vi "Bump Turret Az.vi"() -> ()   [LabVIEW 2016]
panel:
  in  "D-Pad":T1(radio)
  in  "reset":bool
  out "offset":dbl
  out "arctan(x)":dbl
  in  "D":dbl
  in  "d":dbl
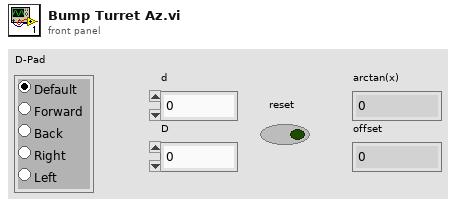
[diagram p1: front panel]
types:
  T1 = enum32{"Default", "Radio Selection 2", "Radio Selection 4", "Radio Selection 3", "Radio Selection 5"}
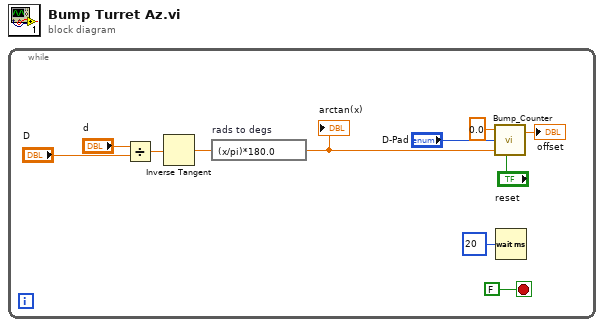
[diagram p0: block diagram]
diagram:
  n1 = while {
    stop <- FALSE stop-if-true
    n2 = Divide(x="d", y="D") -> (x/y=w10:dbl)
    n3 = Inverse Tangent(1:w10) -> (0:w7:dbl)
    n4 = expression code="(x/pi)*180.0" "rads to degs"(w7) -> (w4:dbl)
    "arctan(x)" <- w4
    n5 = call <userlib>:"Bump_Counter.vi"("ref"=0.0, "D-Pad"="D-Pad", "quanta"=w4, "reset"="reset") -> ("out"=→"offset":dbl)  [unwired: 2 in]
    n6 = Wait (ms)(milliseconds to wait=u32 20) -> ()  [unwired: 1 out]
  }
